vi "Sacn Engine Test.vi"   [LabVIEW 2021]
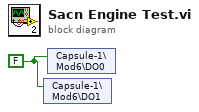
[diagram p0: block diagram]
diagram:
  w1 = FALSE ("DO0")
  n1 = shared-variable "Capsule-1\\Mod6\\DO1"(w1) -> ()  [unwired: 1 in, 1 out]
  n2 = shared-variable "Capsule-1\\Mod6\\DO0"(w1) -> ()  [unwired: 1 in, 1 out]
